vi "Navi R&L ENC Avg.vi"(1 "encoder step sub vi input":dbl[](array[numeric]), 8 "Reset X Y":dbl=1.0) -> (15 "encoder step sub vi output":dbl[](array[numeric]))   [LabVIEW 2015]
panel:
  out "Avg Right Dist. New":dbl
  out "Avg Left Dist. New":dbl
  out "distance step":dbl
  out "Avg Left Step":dbl
  out "Avg Right Step":dbl
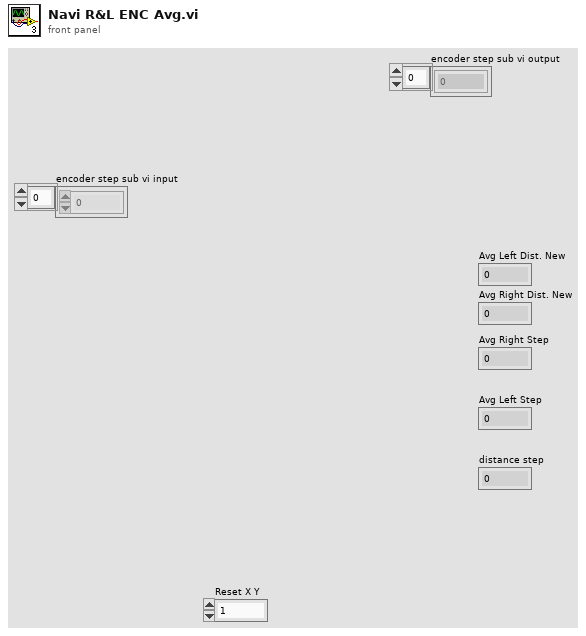
[diagram p1: front panel]
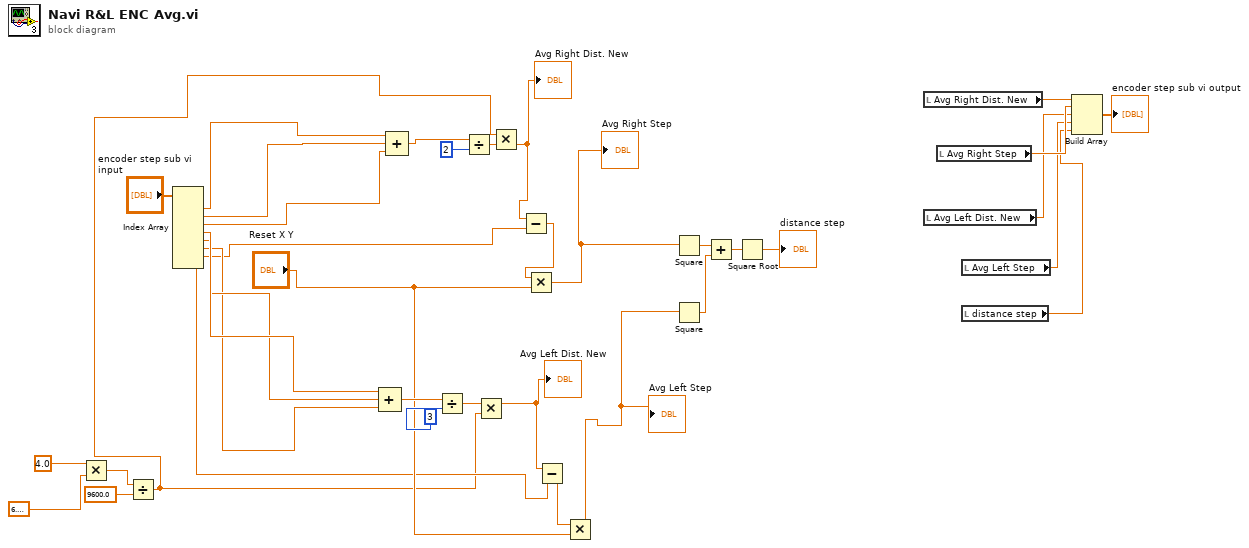
[diagram p0: block diagram]
diagram:
  n1 = Multiply(x=4.0, y=6.283185307179586) -> (x*y=w4:dbl)
  n2 = Divide(x=w4, y=9600.0) -> (x/y=w1:dbl)
  n3 = Index Array(array="encoder step sub vi input") -> (element #1=w26:dbl, element #2=w25:dbl, element #3=w24:dbl, element #4=w23:dbl, element #5=w22:dbl, element #6=w20:dbl, element #7=w19:dbl, element #8=w18:dbl)  [unwired: 8 in]
  n4 = Compound Arithmetic op=ADD(w23, w22, w20) -> (w35:dbl)
  n5 = Compound Arithmetic op=ADD(w26, w25, w24) -> (w37:dbl)
  n6 = Divide(x=w35, y=3) -> (x/y=w8:dbl)
  n7 = Divide(x=w37, y=2) -> (x/y=w17:dbl)
  n8 = Multiply(x=w8, y=w1) -> (x*y=w3:dbl)
  "Avg Left Dist. New" <- w3
  n9 = Multiply(x=w1, y=w17) -> (x*y=w2:dbl)
  "Avg Right Dist. New" <- w2
  n10 = Subtract(x=w2, y=w19) -> (x-y=w28:dbl)
  n11 = Multiply(x=w28, y="Reset X Y") -> (x*y=w16:dbl)
  "Avg Right Step" <- w16
  n12 = Subtract(x=w3, y=w18) -> (x-y=w27:dbl)
  n13 = Multiply(x=w27, y="Reset X Y") -> (x*y=w15:dbl)
  "Avg Left Step" <- w15
  n14 = Square(x=w16) -> (x^2=w31:dbl)
  n15 = Square(x=w15) -> (x^2=w30:dbl)
  n16 = Add(x=w31, y=w30) -> (x+y=w32:dbl)
  n17 = Square Root(x=w32) -> (sqrt(x)=→"distance step":dbl)
  n18 = local read "Avg Right Dist. New"() -> (w14:dbl)
  n19 = local read "Avg Left Dist. New"() -> (w12:dbl)
  n20 = local read "Avg Right Step"() -> (w13:dbl)
  n21 = local read "Avg Left Step"() -> (w11:dbl)
  n22 = local read "distance step"() -> (w10:dbl)
  n23 = Build Array(w14, w13, w12, w11, w10) -> (→"encoder step sub vi output":dbl[])
